vi "GenerateAlphabetArray.vi"() -> (0 "Array":string[](array[string]))   [LabVIEW 2024]
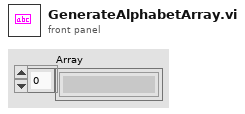
[diagram p1: front panel]
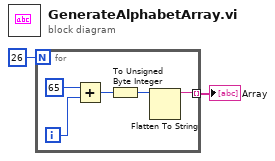
[diagram p0: block diagram]
diagram:
  n1 = for {
    N: 26 -> [_]
    tunnel: [w3] -> w1 mode=indexing
    i -> [w7]
    n2 = Add(x=65, y=w7) -> (x+y=w5:i32)
    n3 = To Unsigned Byte Integer(number=w5) -> (unsigned 8bit integer=w4:u8)
    n4 = Flatten To String(anything=w4) -> (data string=w3:string)  [unwired: 3 in, 2 out]
  }
  "Array" <- w1
